vi "test_RefnumName.vi"() -> ()   [LabVIEW 2013]
uses:
  source/TypeDescriptor/TypeDescriptor_GetPString.vi
  source/TypeDescriptor/OpenDescriptor.lvlib
panel:
  out "Event Class":string[](array[string])
  out "element names":string[](array[string])
  out "data string":string
  out "Class":u8[](array[numeric]) format="%.0x"
  out "Menu":u8[](array[numeric]) format="%.0x"
  out "Event Registration (2 Events)":u8[](array[numeric]) format="%.0x"
  out "AppRef":u8[](array[numeric]) format="%.0x"
  out "subtype":i16 format="%.0x"
  out "DAQmx":u8[](array[numeric]) format="%.0x"
  out "*(type *) &x":string
  out "VISA Resource":u8[](array[numeric]) format="%.0x"
  out "Occurence":u8[](array[numeric]) format="%.0x"
  out "Network Stream":u8[](array[numeric]) format="%.0x"
  out "name":string
  out "Queue":u8[](array[numeric]) format="%.0x"
  out "Notifier":u8[](array[numeric]) format="%.0x"
  out "Semaphore":u8[](array[numeric]) format="%.0x"
  out "Queue Complex":u8[](array[numeric]) format="%.0x"
  out "VIRef":u8[](array[numeric]) format="%.0x"
  # "REF"
  # "VI REF"
  # "size"
  # "types: \nx08 = VIReference\nx12 = Queue\nx01 = Semaphore\nx11 = Notifier"
  # "size"
  # "named"
  # "ref"
  # "REF"
  # "size"
  # "APPREF"
  # "size"
  # "named"
  # "ref"
  # "QUEUE"
  # "size"
  # "named"
  # "# units"
  # "unit type"
  # "unit type"
  # "exponent"
  # "exponent"
  # "unit type"
  # "exponent"
  # "Extended-Precision Complex Physical Quantity"
  # "size"
  # "named"
  # "ref"
  # "size"
  # "named"
  # "SEMAPHORE"
  # "Enumerated 16-bit Integer"
  # "size"
  # "named"
  # "ref"
  # "size"
  # "named"
  # "Nb of\nElements"
  # "NOTIFIER"
  # "Enumerated 8-bit Integer"
  # "size"
  # "named"
  # "ref"
  # "QUEUE"
  # "String"
  # "STREAM"
  # "OCCURENCE"
  # "VISA RSC"
  # "DAQmx"
  # "MENU"
  # "size = 64 (x40)           Refnum\n             named (x40)    (0x70)"
  # "subtype\nRegRef"
  # "size = 32 (x20)           # elem\n             named (x00)    (1)"
  # "type\n(0x08)"
  # "label size:\n7"
  # "size = 20 (x14)           Refnum\n             named (x40)    (0x70)"
  # "T"
  # "h"
  # "i"
  # "s"
  # "[SP]"
  # "V"
  # "I"
  # "First Element"
  # "EventRefnum (x70 = refnum; x0008 = Generic Ref)"
  # "size = 10 (xA)"
  # "size = 10 (xA)"
  # "First Element"
  # "Second Element"
  # "# element"
  # "Event DataType (x3 = I32)"
  # "Event DataType (x21 = Boolean)"
  # "size = 22 (x0016)\nnamed (x40)"
  # "size = 24 (x0018)\nnamed (x40)"
  # "EventRefnum (x70 = refnum; x0019 = Event Ref)"
  # "EventRefnum (x70 = refnum; x0019 = Event Ref)"
  # "subtype\nRegRef"
  # "size = 66 (x0042)\nunnamed (x00)"
  # "EventRegistration (x0017 = Registration Reference Subtype)"
  # "size = 80 (x50)\nnamed (x40)"
  # "Reference (x70 = refnum)"
  # "Class\nsubtype"
  # "size"
  # "EventLabel (Event)"
  # "size"
  # "Class Path (LabVIEW Object)"
  # "size"
  # "Name (Refnum)"
  # "size"
  # "TypeLabel (bool)"
  # "size"
  # "EventLabel (Event2)"
  # "size"
  # "TypeLabel (test)"
  # "size"
  # "EventLabel (Event)"
  # "size"
  # "Name (Refnum)"
  # "size"
  # "pad"
  # "Name (Refnum)"
  # "size"
  # "pad"
  # "Name (Refnum)"
  # "size"
  # "pad"
  # "Name (Refnum)"
  # "size"
  # "Type (Instr)"
  # "size"
  # "pad"
  # "Name (Refnum)"
  # "size"
  # "pad"
  # "Name (Refnum)"
  # "size"
  # "DataExcahnge Type (NetworkStream)"
  # "size"
  # "pad"
  # "Subtype (DataExchange)"
  # "size"
  # "pad"
  # "Name (Refnum)"
  # "size"
  # "term"
  # "Element Name (Complex)"
  # "size"
  # "pad"
  # "Name (Refnum)"
  # "size"
  # "term"
  # "Name (Refnum)"
  # "size"
  # "Element Name (Complex)"
  # "size"
  # "Element Name (Item3A)"
  # "size"
  # "Element Name (Item2)"
  # "size"
  # "Element Name (Item1)"
  # "size"
  # "Enum Label (semaphore)"
  # "size"
  # "Item Name (semaphore)"
  # "size"
  # "pad"
  # "Name (Refnum)"
  # "size"
  # "Element Name (Complex)"
  # "size"
  # "pad"
  # "Name (Refnum)"
  # "size"
  # "pad"
  # "Name (Refnum)"
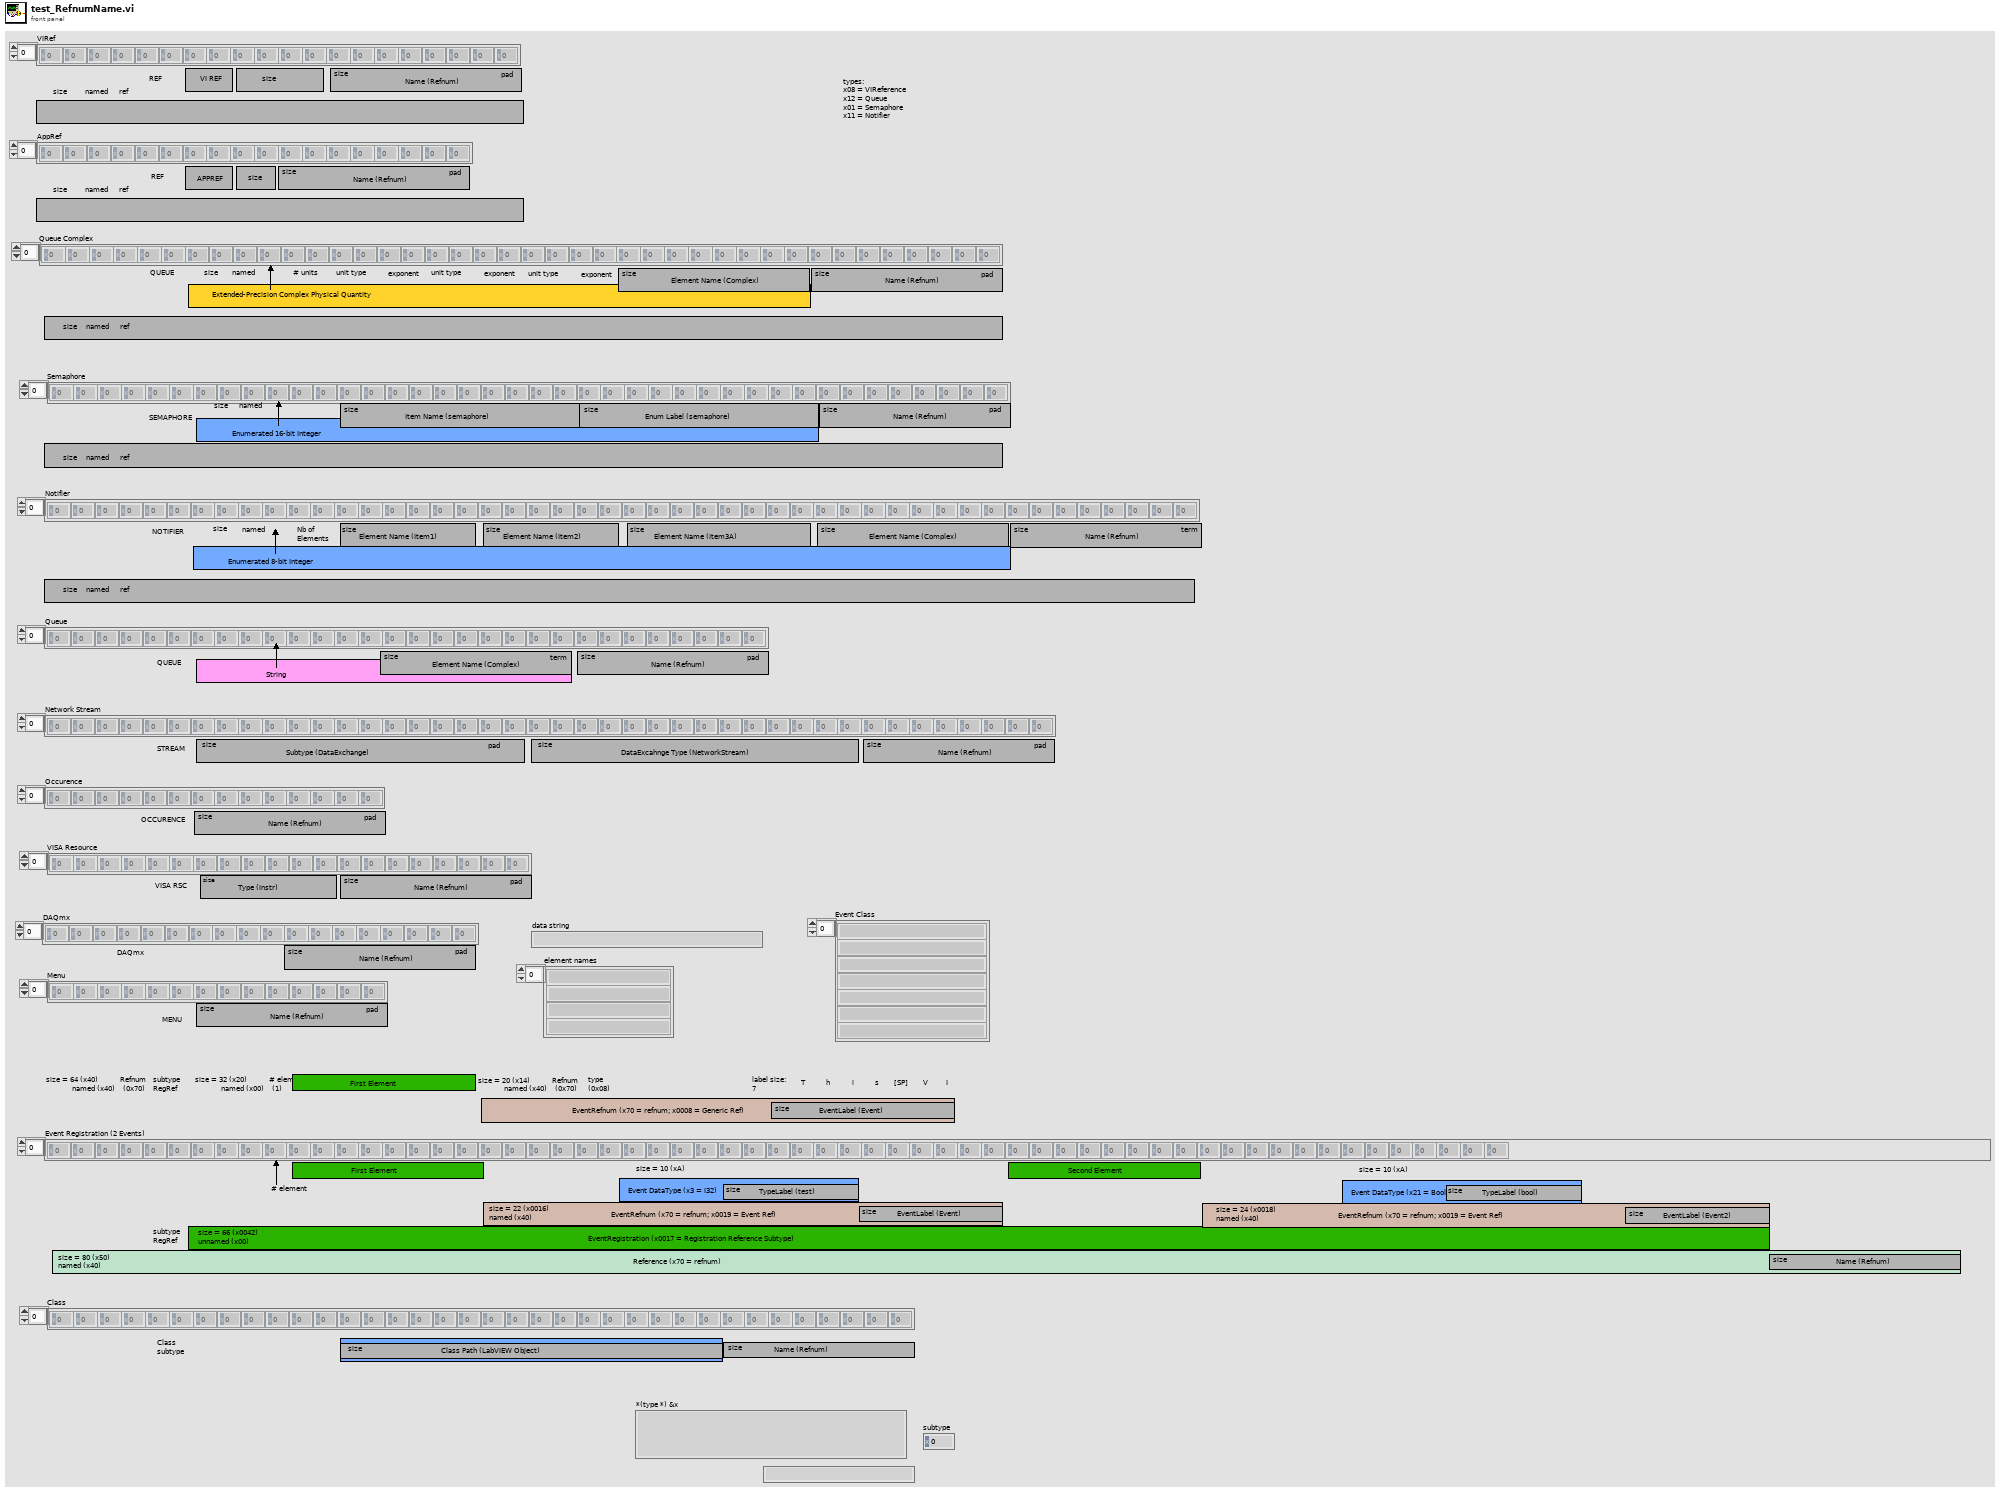
[diagram p1: front panel]
types:
  T1 = typedef "Rendezvous RefNum" = refnum<k1>
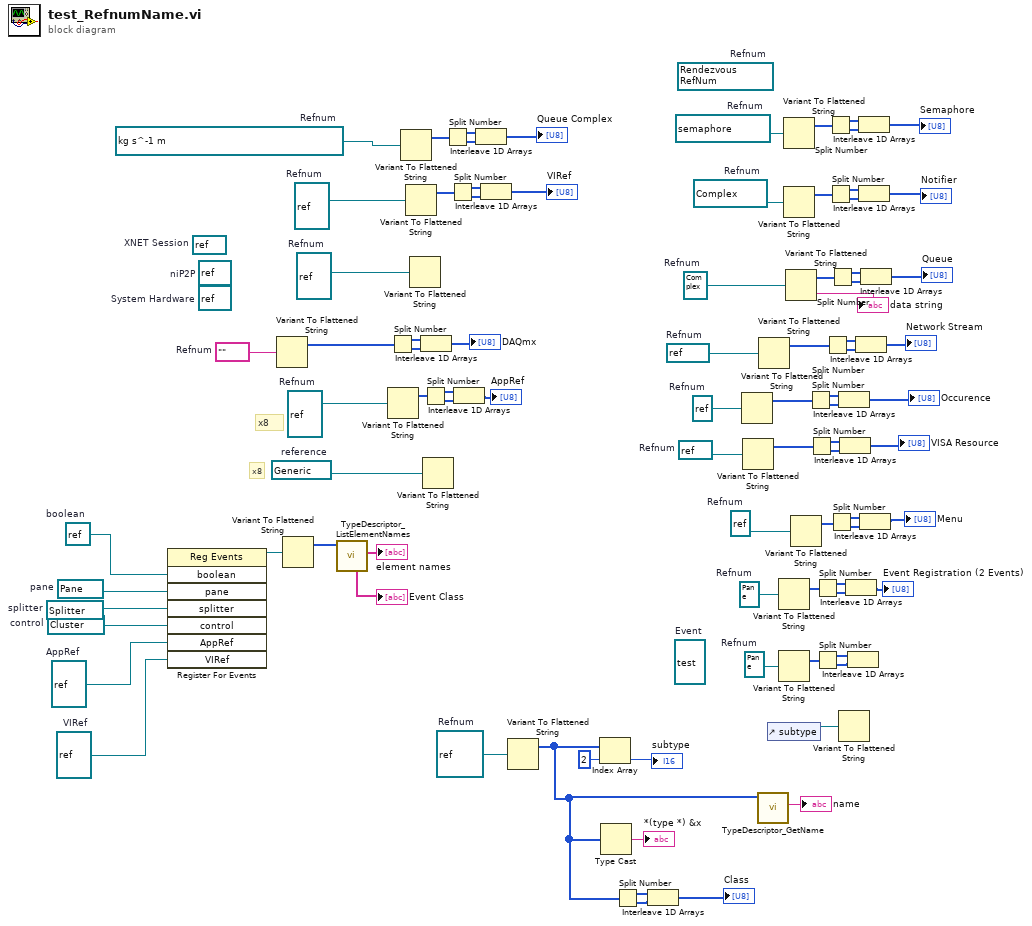
[diagram p0: block diagram]
diagram:
  w1 = refnum<vi> refnum  # VIRef
  w2 = refnum<vi> refnum  # AppRef
  w3 = refnum<vi> refnum  # control
  w7 = refnum<user-event> refnum  # boolean
  w4 = refnum<vi> refnum  # splitter
  w5 = refnum<vi> refnum  # pane
  w14 = refnum<class> refnum  # Refnum
  (unwired) refnum<user-event> refnum  # Event
  w23 = refnum<event-registration> refnum  # Refnum
  w21 = refnum<event-registration> refnum  # Refnum
  w24 = refnum<k9> refnum  # Refnum
  w29 = refnum<vi> refnum  # Refnum
  w13 = refnum<vi> refnum  # reference
  (unwired) refnum<k20> refnum  # System Hardware
  (unwired) refnum<k20> refnum  # niP2P
  (unwired) refnum<k21> refnum  # XNET Session
  w40 = tag ""  # Refnum
  w45 = refnum<visa-resource-name> refnum  # Refnum
  w51 = refnum<k4> refnum  # Refnum
  w56 = refnum<k21> refnum  # Refnum
  (unwired) T1 refnum items=["rendezvous"]  # Refnum
  w61 = refnum<vi> refnum  # Refnum
  w63 = refnum<queue> refnum  # Refnum
  w76 = refnum<notifier> refnum items=["Item1", "Item2", "Item3A"]  # Refnum
  w71 = refnum<k1> refnum items=["semaphore"]  # Refnum
  w70 = refnum<vi> refnum  # Refnum
  w85 = refnum<queue> refnum  # Refnum
  # "x8"
  # "x8"
  n1 = register-events(w7, w5, w4, w3, w2, w1) -> (reference out=w6:refnum<event-registration>)  [unwired: 2 in, 1 out]
  n2 = Variant To Flattened String(Variant=w40) -> (1:w44:i16[])  [unwired: 1 out]
  n3 = Variant To Flattened String(Variant=w6) -> (1:w10:i16[])  [unwired: 1 out]
  n4 = call "TypeDescriptor_ListElementNames.vi"("type descriptor"=w10) -> ("element names"=→"element names":string[], "Event Class"=→"Event Class":string[])  [unwired: 7 in, 2 out]
  n5 = Split Number(x=w44) -> (hi(x)=w42:u8[], lo(x)=w43:u8[])
  n6 = Variant To Flattened String(Variant=w29) -> (1:w34:i16[])  [unwired: 1 out]
  n7 = Variant To Flattened String(Variant=w85) -> (1:w66:i16[])  [unwired: 1 out]
  n8 = Variant To Flattened String(Variant=w70) -> (1:w62:i16[])  [unwired: 1 out]
  n9 = Variant To Flattened String(Variant=w61) -> ()  [unwired: 2 out]
  n10 = Interleave 1D Arrays(w42, w43) -> (→"DAQmx":u8[])
  n11 = Split Number(x=w34) -> (hi(x)=w37:u8[], lo(x)=w36:u8[])
  n12 = Variant To Flattened String(Variant=w13) -> ()  [unwired: 2 out]
  n13 = Split Number(x=w66) -> (hi(x)=w87:u8[], lo(x)=w86:u8[])
  n14 = Split Number(x=w62) -> (hi(x)=w82:u8[], lo(x)=w83:u8[])
  n15 = Interleave 1D Arrays(w37, w36) -> (→"AppRef":u8[])
  n16 = Interleave 1D Arrays(w87, w86) -> (→"Queue Complex":u8[])
  n17 = Interleave 1D Arrays(w82, w83) -> (→"VIRef":u8[])
  n18 = Variant To Flattened String(Variant=w14) -> (1:w16:i16[])  [unwired: 1 out]
  n19 = Index Array(array=w16, index=2) -> (element=→"subtype":i16)
  n20 = Type Cast(x=w16) -> (*(type *) &x=→"*(type *) &x":string)  [unwired: 1 in]
  n21 = Split Number(x=w16) -> (hi(x)=w17:u8[], lo(x)=w18:u8[])
  n22 = Interleave 1D Arrays(w17, w18) -> (→"Class":u8[])
  n23 = Variant To Flattened String(Variant=w51) -> (1:w53:i16[])  [unwired: 1 out]
  n24 = Variant To Flattened String(Variant=w45) -> (1:w47:i16[])  [unwired: 1 out]
  n25 = call "TypeDescriptor_GetName.vi"("type descriptor"=w16) -> ("name"=→"name":string)  [unwired: 8 in, 2 out]
  n26 = Variant To Flattened String(Variant=w56) -> (1:w57:i16[])  [unwired: 1 out]
  n27 = control-ref of="subtype"() -> (w12:refnum<vi>)
  n28 = Variant To Flattened String(Variant=w23) -> (1:w30:i16[])  [unwired: 1 out]
  n29 = Variant To Flattened String(Variant=w21) -> (1:w22:i16[])  [unwired: 1 out]
  n30 = Variant To Flattened String(Variant=w71) -> (1:w65:i16[])  [unwired: 1 out]
  n31 = Variant To Flattened String(Variant=w76) -> (1:w67:i16[])  [unwired: 1 out]
  n32 = Variant To Flattened String(Variant=w63) -> (data string=→"data string":string, 1:w64:i16[])
  n33 = Variant To Flattened String(Variant=w24) -> (1:w25:i16[])  [unwired: 1 out]
  n34 = Split Number(x=w53) -> (hi(x)=w54:u8[], lo(x)=w55:u8[])
  n35 = Split Number(x=w47) -> (hi(x)=w50:u8[], lo(x)=w49:u8[])
  n36 = Split Number(x=w30) -> (hi(x)=w31:u8[], lo(x)=w32:u8[])
  n37 = Split Number(x=w22) -> (hi(x)=w20:u8[], lo(x)=w19:u8[])
  n38 = Split Number(x=w57) -> (hi(x)=w60:u8[], lo(x)=w59:u8[])
  n39 = Split Number(x=w65) -> (hi(x)=w80:u8[], lo(x)=w79:u8[])
  n40 = Split Number(x=w67) -> (hi(x)=w77:u8[], lo(x)=w78:u8[])
  n41 = Split Number(x=w25) -> (hi(x)=w28:u8[], lo(x)=w27:u8[])
  n42 = Split Number(x=w64) -> (hi(x)=w72:u8[], lo(x)=w73:u8[])
  n43 = Interleave 1D Arrays(w54, w55) -> (→"Occurence":u8[])
  n44 = Variant To Flattened String(Variant=w12) -> ()  [unwired: 2 out]
  n45 = Interleave 1D Arrays(w50, w49) -> (→"VISA Resource":u8[])
  n46 = Interleave 1D Arrays(w31, w32) -> (→"Event Registration (2 Events)":u8[])
  n47 = Interleave 1D Arrays(w20, w19) -> ()  [unwired: 1 out]
  n48 = Interleave 1D Arrays(w60, w59) -> (→"Network Stream":u8[])
  n49 = Interleave 1D Arrays(w80, w79) -> (→"Semaphore":u8[])
  n50 = Interleave 1D Arrays(w77, w78) -> (→"Notifier":u8[])
  n51 = Interleave 1D Arrays(w28, w27) -> (→"Menu":u8[])
  n52 = Interleave 1D Arrays(w72, w73) -> (→"Queue":u8[])
